vi "Rohde & Schwarz VNA Read Trace Status.vi"(4 "Trace":i32=1 min=1 max=99 step=1 format="%#_2f", 6 "Channel":i32=1 min=1 max=99 step=1 format="%#_2f", 7 "Rohde & Schwarz VNA":T1, 8 "error in (no error)":errorcluster, 11 "VISA Resource Name":refnum<visa-resource-name>) -> (0 "error out":errorcluster, 2 "On?":bool, 3 "dup VISA Resource Name":refnum<visa-resource-name>)   [LabVIEW 2011]
uses:
  TypeDefs/Rohde & Schwarz VNA Instrument Info.ctl
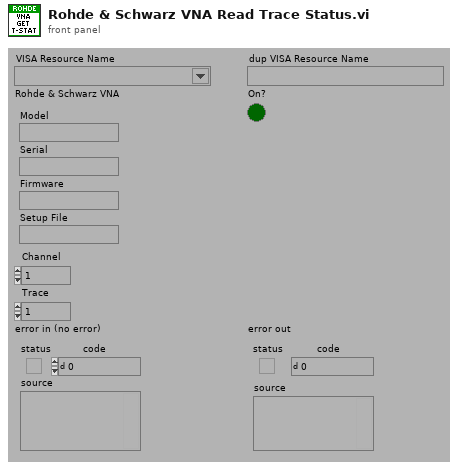
[diagram p1: front panel]
types:
  T1 = typedef "Rohde & Schwarz VNA Instrument Info.ctl" = cluster{"Model":string, "Serial":string, "Firmware":string, "Setup File":string}
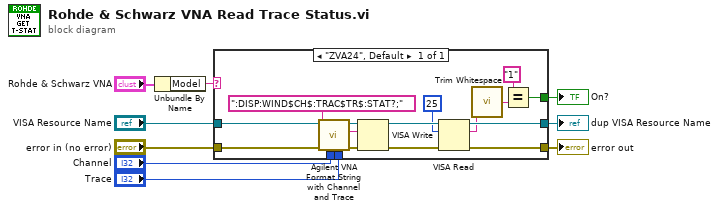
[diagram p0: block diagram]
diagram:
  n1 = Unbundle By Name("Rohde & Schwarz VNA") -> ("Model"=w1:string)
  n2 = case shown="\"ZVA24\", Default" w1 {
    tunnel: "VISA Resource Name" -> [w24]
    tunnel: "error in (no error)" -> [w23]
    tunnel: [w20] -> w7
    tunnel: [w19] -> w6
    tunnel: [w14] -> w5
    tunnel: "Channel" -> [w11]
    tunnel: "Trace" -> [w10]
    frame "ZVA24", Default {
      n3 = call "Agilent VNA Format String with Channel and Trace.vi"("Trace"=w10, "Channel"=w11, "String"=":DISP:WIND$CH$:TRAC$TR$:STAT?;" ("write buffer")) -> ("String Out"=w12:string)  [unwired: 6 out]
      n4 = VISA Write(VISA resource name=w24, write buffer=w12, error in (no error)=w23) -> (VISA resource name out=w21:refnum<visa-resource-name>, error out=w22:errorcluster)  [unwired: 1 out]
      n5 = VISA Read(VISA resource name=w21, byte count=u32 25, error in (no error)=w22) -> (VISA resource name out=w20:refnum<visa-resource-name>, read buffer=w17:string, error out=w19:errorcluster)  [unwired: 1 out]
      n6 = call <vilib>:"Trim Whitespace.vi"("string"=w17) -> ("trimmed string"=w16:string)  [unwired: 1 in]
      n7 = Equal?(x="1", y=w16) -> (x = y?=w14:bool)
    }
  }
  "dup VISA Resource Name" <- w7
  "error out" <- w6
  "On?" <- w5
